vi "Trace.vi"(7 "Trace Level":T1(ring)=enum."Debug", 8 "error in (no error)":errorcluster, 9 "Command Message":string, 10 "Command Action":string, 11 "Command Actor in":refnum<class "Command Actor.lvclass">) -> (0 "error out":errorcluster, 3 "Command Actor out":refnum<class "Command Actor.lvclass">)   [LabVIEW 2014, in "Robot Actor Framework.lvlib" / "Command Actor.lvlib" / "Command Actor.lvclass"]
uses:
  Command Actor.lvclass
  Trace/Trace Class/Trace.lvclass
  Command Actor.lvclass/Command Actor.ctl
  System Actor/System Actor Messages/Record Trace Msg/Record Trace Msg.lvclass/Record Trace Msg.ctl
  <vilib>/ActorFramework/Message Enqueuer/Message Enqueuer.lvclass/Message Enqueuer.ctl
  <vilib>/ActorFramework/Message Enqueuer/Enqueue.vi
  Utilities/Call Stack to String.vi
  <vilib>/ActorFramework/Message Priority Queue/Priority Enqueue.vi
  System Actor/System Actor Messages/Record Trace Msg/Record Trace Msg.lvclass
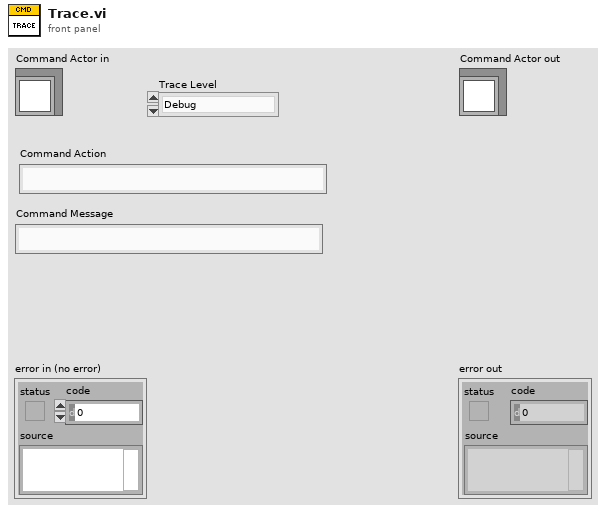
[diagram p1: front panel]
types:
  T1 = enum16{"Critical", "Error", "Warning", "Informational", "Debug"}
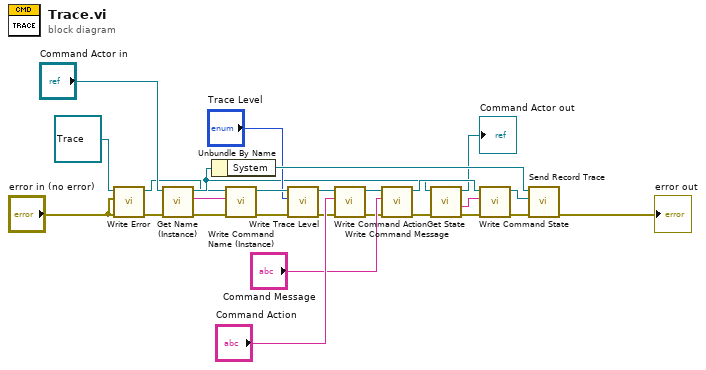
[diagram p0: block diagram]
diagram:
  n1 = call-dynamic "Write Error.vi"("error in (no error)"="error in (no error)", "Error"="error in (no error)", "Trace in"=refnum<class "Trace.lvclass"> refnum ("Robot Actor Framework.lvlib:Trace.lvlib:Trace.lvclass")) -> ("error out"=w1:errorcluster, "Trace out"=w3:refnum<class "Trace.lvclass">)  [unwired: 7 in]
  n2 = call-dynamic "Get Name (Instance).vi"("error in (no error)"=w1, "Command Actor in"="Command Actor in") -> ("error out"=w12:errorcluster, "Name (Instance)"=w25:string, "Command Actor out"=w15:refnum<class "Command Actor.lvclass">)  [unwired: 7 in]
  n3 = Unbundle By Name(w15) -> ("System"=w24:refnum<class "Message Enqueuer.lvclass">)
  n4 = call-dynamic "Write Command Name (Instance).vi"("error in (no error)"=w12, "Command Name (Instance)"=w25, "Trace in"=w3) -> ("error out"=w11:errorcluster, "Trace out"=w23:refnum<class "Trace.lvclass">)  [unwired: 7 in]
  n5 = call-dynamic "Write Trace Level.vi"("error in (no error)"=w11, "Trace Level"="Trace Level", "Trace in"=w23) -> ("error out"=w10:errorcluster, "Trace out"=w22:refnum<class "Trace.lvclass">)  [unwired: 7 in]
  n6 = call-dynamic "Write Command Action.vi"("error in (no error)"=w10, "Command Action"="Command Action", "Trace in"=w22) -> ("error out"=w9:errorcluster, "Trace out"=w21:refnum<class "Trace.lvclass">)  [unwired: 7 in]
  n7 = call-dynamic "Write Command Message.vi"("error in (no error)"=w9, "Command Message"="Command Message", "Trace in"=w21) -> ("error out"=w8:errorcluster, "Trace out"=w17:refnum<class "Trace.lvclass">)  [unwired: 7 in]
  n8 = call-dynamic "Get State.vi"("error in (no error)"=w8, "Command in"=w15) -> ("error out"=w7:errorcluster, "Command State String"=w13:string, "Command out"=→"Command Actor out":refnum<class "Command Actor.lvclass">)  [unwired: 7 in]
  n9 = call-dynamic "Write Command State.vi"("error in (no error)"=w7, "Command State"=w13, "Trace in"=w17) -> ("error out"=w6:errorcluster, "Trace out"=w16:refnum<class "Trace.lvclass">)  [unwired: 7 in]
  n10 = call "Send Record Trace.vi"("error in (no error)"=w6, "Trace"=w16, "Message Enqueuer"=w24) -> ("error out"=→"error out":errorcluster)  [unwired: 7 in, 1 out]
